vi "Write TDMS File.vi"(8 "error in":errorcluster, 10 "Data":dbl[][](array[numeric]) format="%0.2f", 11 "File Path":path) -> (0 "error out":errorcluster)   [LabVIEW 2021]
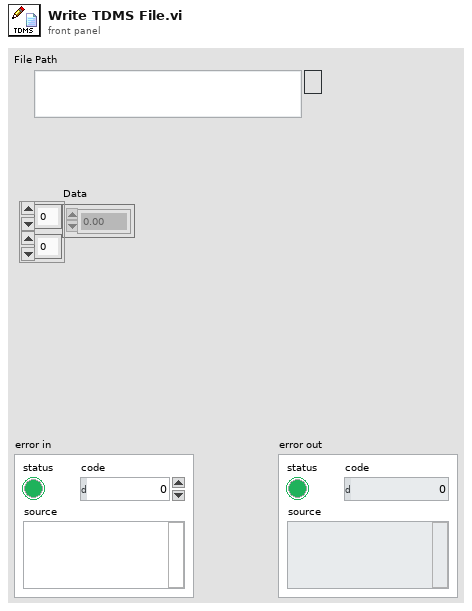
[diagram p1: front panel]
types:
  T1 = enum16{"open", "open or create", "create or replace", "create", "open (read-only)"}
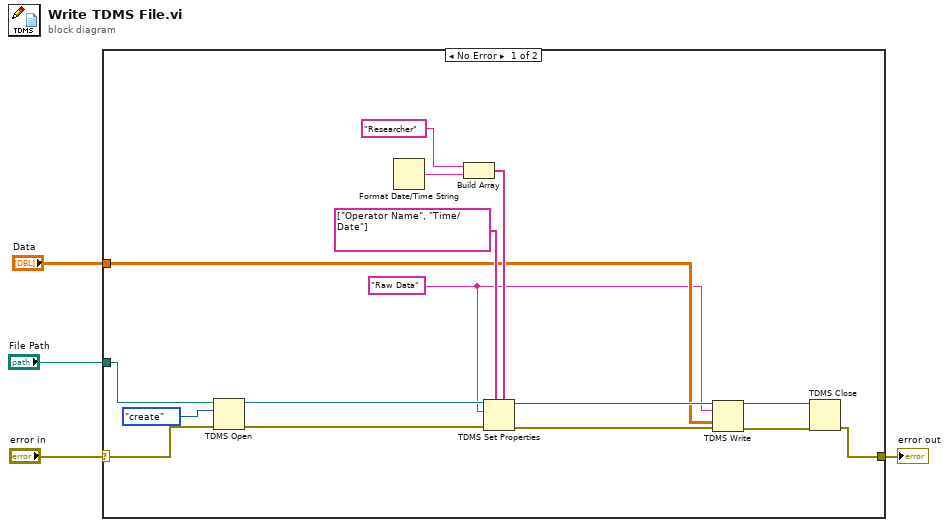
[diagram p0: block diagram]
diagram:
  n1 = case shown="No Error" "error in" {
    selector: "error in" -> [w20 w21]
    tunnel: [w9 w21] -> w3
    tunnel: "File Path" -> [w19 _]
    tunnel: "Data" -> [w6 _]
    frame No Error {
      w5 = "Raw Data"
      n2 = TDMS Open(8:w20, 10:T1."create" ("operation (0:open)"), 11:w19) -> (0:w17:errorcluster, 3:w18:refnum<k34>)  [unwired: 4 in]
      n3 = Format Date/Time String() -> (date/time string=w11:string)  [unwired: 3 in]
      n4 = Build Array("Researcher", w11) -> (w7:string[])
      n5 = TDMS Set Properties(5:w7, 7:string[] ["Operator Name", "Time/Date"], 8:w17, 10:w5, 11:w18) -> (0:w14:errorcluster, 3:w16:refnum<k34>)  [unwired: 1 in, 2 out]
      n6 = TDMS Write(0:w16, 5:w5, 9:w6, 11:w14) -> (4:w15:refnum<k34>, 15:w13:errorcluster)  [unwired: 2 in, 2 out]
      n7 = TDMS Close(8:w13, 11:w15) -> (0:w9:errorcluster)  [unwired: 1 out]
    }
    frame Error {
    }
  }
  "error out" <- w3
